vi "point-by-point speed and angle original.vi"(6 "encoders offset":u32 caption="encoder offset @ 1Hz (ticks)", 8 "speed history in":u32[](array[numeric])=[0, 0, 0, 0, 0, 0, 0, 0, 0, 0, 0, 0, 0, 0, 0, 0, 0, 0, 0, 0, 0, 0, 0, 0, 0, 0, 0, 0, 0, 0, 0, 0, 0, 0, 0, 0, 0, 0, 0, 0], 10 "angle pulse":u32, 11 "speed pulse":u32) -> (0 "speed history out":u32[](array[numeric]), 2 "calculated angle (degrees)":sgl, 3 "calculated speed (Hz)":sgl, 4 "measured encoder delta":sgl)   [LabVIEW 2018]
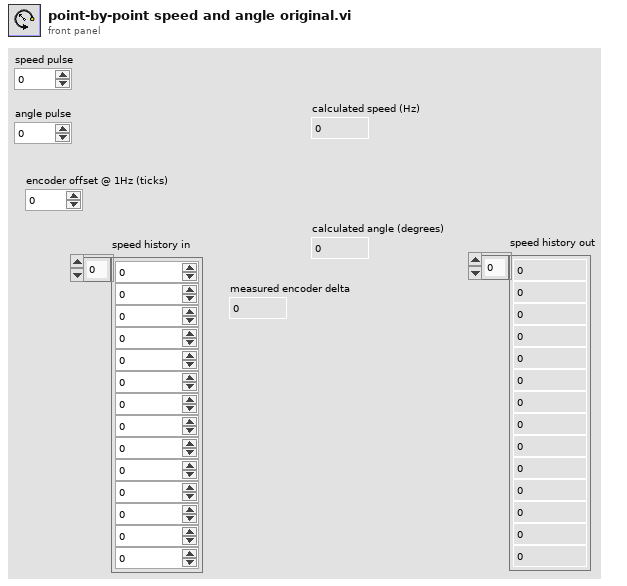
[diagram p1: front panel]
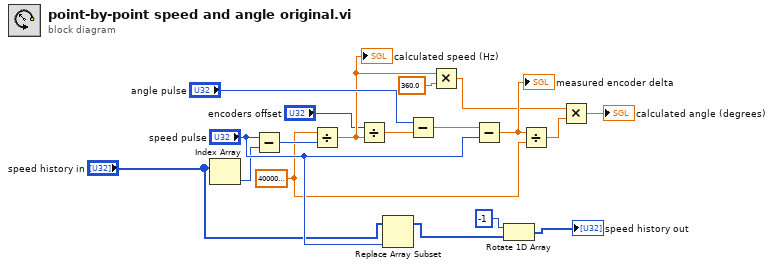
[diagram p0: block diagram]
diagram:
  w10 = sgl 40000000.0 ("64bit integer")
  n1 = Index Array(array="speed history in") -> (element=w16:u32)  [unwired: 1 in]
  n2 = Subtract(x="speed pulse", y=w16) -> (x-y=w14:u32)
  n3 = Divide(x=w10, y=w14) -> (x/y=w5:sgl)
  "calculated speed (Hz)" <- w5
  n4 = Divide(x="encoders offset", y=w5) -> (x/y=w6:sgl)
  n5 = Replace Array Subset(array="speed history in", new element="speed pulse") -> (w2:u32[])  [unwired: 1 in]
  n6 = Subtract(x="angle pulse", y=w6) -> (x-y=w13:sgl)
  n7 = Multiply(x=w5, y=sgl 360.0) -> (x*y=w8:sgl)
  n8 = Subtract(x=w13, y="speed pulse") -> (x-y=w11:sgl)
  "measured encoder delta" <- w11
  n9 = Rotate 1D Array(1:w2, 2:-1 ("n")) -> (0:→"speed history out":u32[])
  n10 = Divide(x=w11, y=w10) -> (x/y=w9:sgl)
  n11 = Multiply(x=w8, y=w9) -> (x*y=→"calculated angle (degrees)":sgl)
